vi "Memory.Pointer.Write Bytes.vi"   [LabVIEW 2016, in "LabVIEW Memory Manager.lvlib" / "Memory.Pointer.lvclass"]
uses:
  Memory.Pointer.lvclass
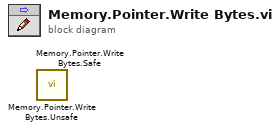
[diagram p0: block diagram]
diagram:
  n1 = call "Memory.Pointer.Write Bytes.Unsafe.vi"() -> ()  [unwired: 8 in, 4 out]
  n2 = call "Memory.Pointer.Write Bytes.Safe.vi"() -> ()  [unwired: 8 in, 4 out]
